vi "IsolarBolaGoleiro.vi"(7 "X goleiro":dbl format="%#_13g", 8 "Y bola":dbl format="%#_13g", 11 "X bola":dbl format="%#_13g") -> (0 "Orientação":dbl format="%#_13g", 2 "Y goleiro":dbl format="%#_13g", 3 "X goleiro":dbl format="%#_13g")   [LabVIEW 2017]
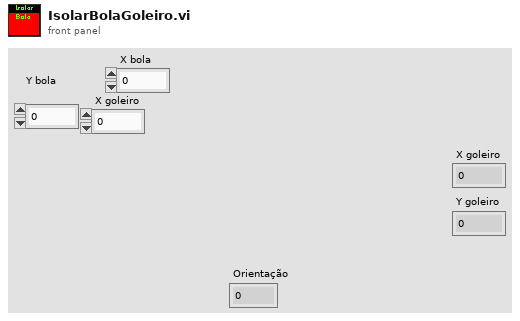
[diagram p1: front panel]
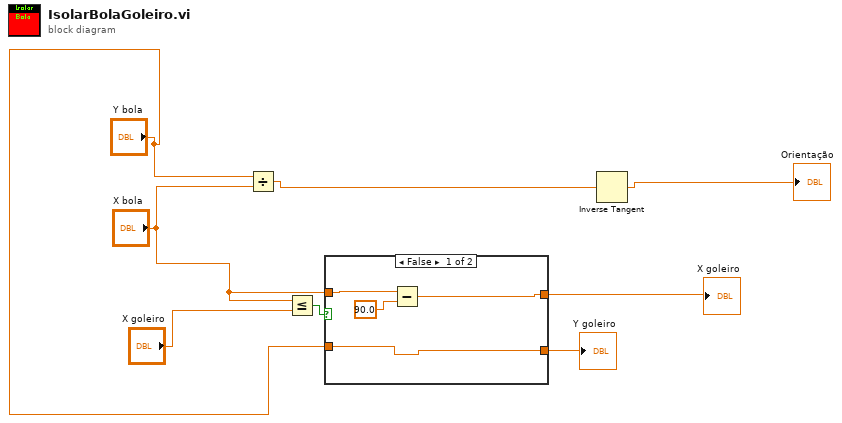
[diagram p0: block diagram]
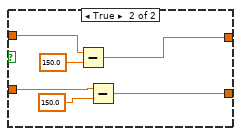
[diagram p2: hidden frame]
diagram:
  n1 = Divide(x="Y bola", y="X bola") -> (x/y=w8:dbl)
  n2 = Less Or Equal?(x="X bola", y="X goleiro") -> (x <= y?=w5:bool)
  n3 = case shown="False" w5 {
    tunnel: "X bola" -> [w12 w18]
    tunnel: [w10 w16] -> w3
    tunnel: "Y bola" -> [w9 w15]
    tunnel: [w9 w13] -> w1
    frame False {
      n4 = Subtract(x=w12, y=90.0 ("x-y")) -> (x-y=w10:dbl)
    }
    frame True {
      n5 = Subtract(x=w18, y=150.0) -> (x-y=w16:dbl)
      n6 = Subtract(x=w15, y=150.0 ("x-y")) -> (x-y=w13:dbl)
    }
  }
  "X goleiro" <- w3
  "Y goleiro" <- w1
  n7 = Inverse Tangent(1:w8) -> (0:→"Orientação":dbl)
